vi "GetSpeedParameters.vi"(8 "error in (no error)":errorcluster, 11 "Channel Config":T2) -> (0 "error out":errorcluster, 3 "nameplate information":T1)   [LabVIEW 2017, in "McsaAnalysisFunctions.lvlib"]
uses:
  <vilib>/addons/InsightCM/Utilities/Analysis/MCSA/McsaAnalysisFunctions.lvlib
  <vilib>/addons/InsightCM/Utilities/Analysis/MCSA/controls/McsaMotor.ctl
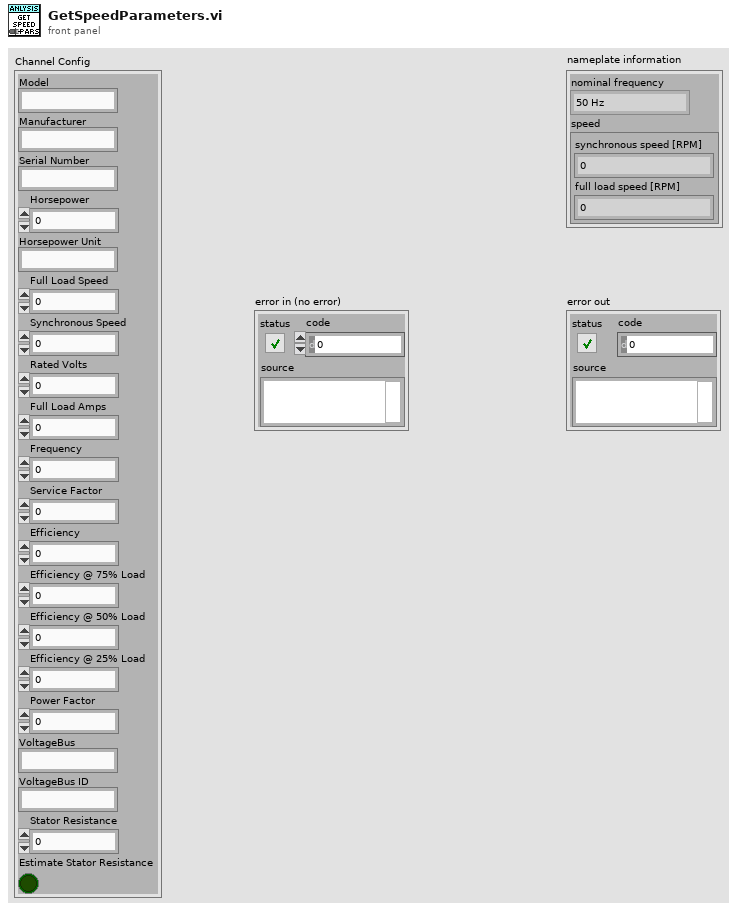
[diagram p1: front panel]
types:
  T1 = cluster{"nominal frequency":enum16{"50 Hz", "60 Hz"}, "speed":cluster{"synchronous speed [RPM]":dbl, "full load speed [RPM]":dbl}}
  T2 = typedef "McsaAnalysisFunctions.lvlib/McsaMotor.ctl" = cluster{"Model":string, "Manufacturer":string, "Serial Number":string, "Horsepower":dbl, "Horsepower Unit":string, "Full Load Speed":dbl, "Synchronous Speed":dbl, "Rated Volts":dbl, "Full Load Amps":dbl, "Frequency":dbl, "Service Factor":dbl, "Efficiency":dbl, "Efficiency @ 75% Load":dbl, "Efficiency @ 50% Load":dbl, "Efficiency @ 25% Load":dbl, "Power Factor":dbl, "VoltageBus":string, "VoltageBus ID":string, "Stator Resistance":dbl, "Estimate Stator Resistance":bool}
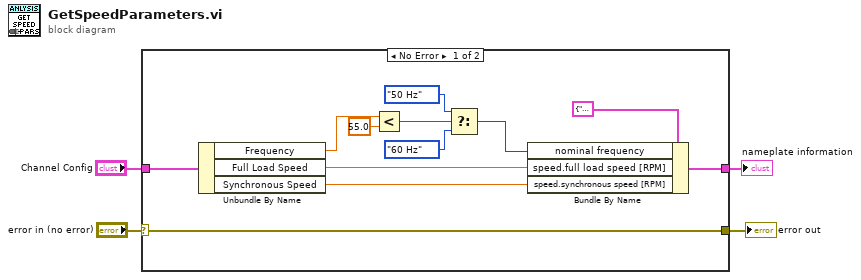
[diagram p0: block diagram]
diagram:
  n1 = case shown="No Error" "error in (no error)" {
    selector: "error in (no error)" -> [w5 w17]
    tunnel: "Channel Config" -> [w16 _]
    tunnel: [w12 _] -> w3
    tunnel: [w5 w17] -> w1
    frame No Error {
      n2 = Unbundle By Name(w16) -> ("Frequency"=w11:dbl, "Full Load Speed"=w14:dbl, "Synchronous Speed"=w13:dbl)
      n3 = Less?(x=w11, y=55.0) -> (x < y?=w9:bool)
      n4 = Select(t=enum16{"50 Hz", "60 Hz"}."50 Hz" ("nominal frequency"), s=w9, f=enum16{"50 Hz", "60 Hz"}."60 Hz" ("nominal frequency")) -> (s? t:f=w8:enum16{"50 Hz", "60 Hz"})
      n5 = Bundle By Name(cluster=T1 {"nominal frequency"=enum."50 Hz", "speed"={"synchronous speed [RPM]"=0.0, "full load speed [RPM]"=0.0}} ("nameplate information"), "nominal frequency"=w8, "speed.full load speed [RPM]"=w14, "speed.synchronous speed [RPM]"=w13) -> (w12:T1)
    }
    frame Error {
    }
  }
  "error out" <- w1
  "nameplate information" <- w3
